vi "(Loop) HVPS_2.vi"   [LabVIEW 2017]
uses:
  Controls/(Ctrl) State_HVPS CMD.ctl
  Variables/(Var) System.vi
  Variables/(Var) Get_HVPS_2.vi
types:
  T1 = typedef "(Ctrl) State_HVPS CMD.ctl" = enum16{"Open", "Rx : V", "Rx : mA", "Rx : State", "Rx : ADC", "Tx : Set V", "Tx : Set mA", "Tx : ON", "Tx : OFF", "Close"}
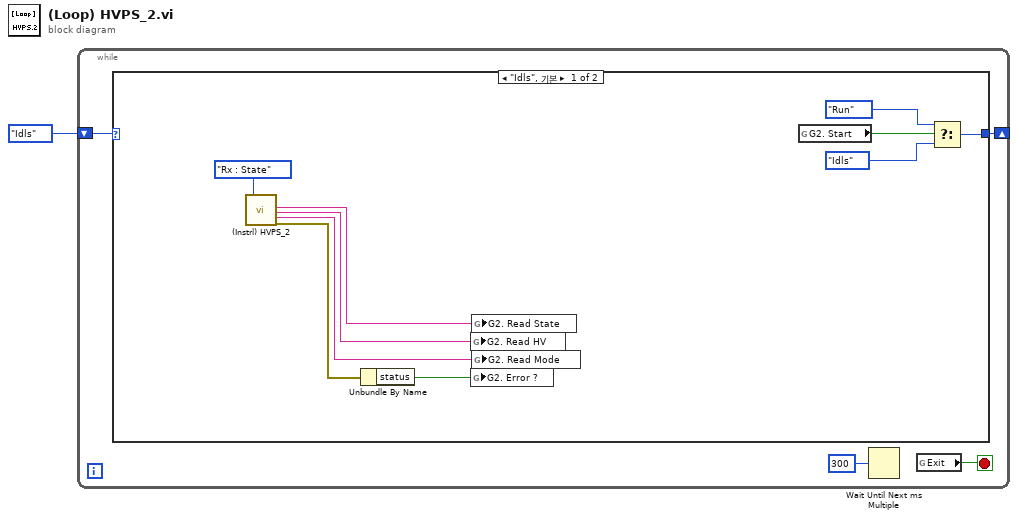
[diagram p0: block diagram]
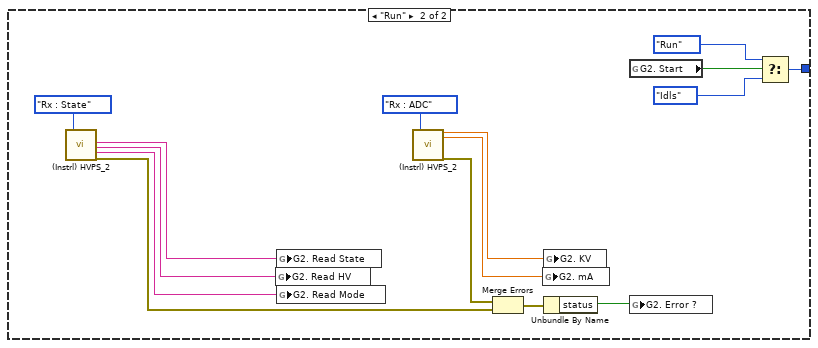
[diagram p2: hidden frame]
diagram:
  n1 = while {
    shift-right: [w2] -> _
    shift-left: enum16{"Init", "Idls", "Run", "Stop", "Close"}."Idls" -> [w4]
    stop <- w5 stop-if-true
    n2 = case shown="\"Idls\", 기본" w4 {
      tunnel: [w11 w27] -> w2
      frame "Idls", Default {
        n3 = call "(Instrl) HVPS_2.vi"("CMD"=(Ctrl)_State_HVPS_CMD."Rx : State" ("State")) -> ("System State"=w10:string, "HV State"=w9:string, "Operation Mode"=w8:string, "error out"=w14:errorcluster)  [unwired: 13 in, 2 out]
        n4 = Unbundle By Name(w14) -> ("status"=w7:bool)
        n5 = global write "(Var) Get_HVPS_2.vi" "G2. Read HV"(w9) -> ()
        n6 = global write "(Var) Get_HVPS_2.vi" "G2. Error ?"(w7) -> ()
        n7 = global write "(Var) Get_HVPS_2.vi" "G2. Read State"(w10) -> ()
        n8 = global write "(Var) Get_HVPS_2.vi" "G2. Read Mode"(w8) -> ()
        n9 = global read "(Var) Get_HVPS_2.vi" "G2. Start"() -> (w6:bool)
        n10 = Select(t=enum16{"Init", "Idls", "Run", "Stop", "Close"}."Run", s=w6, f=enum16{"Init", "Idls", "Run", "Stop", "Close"}."Idls") -> (s? t:f=w11:enum16{"Init", "Idls", "Run", "Stop", "Close"})
      }
      frame "Run" {
        n11 = call "(Instrl) HVPS_2.vi"("CMD"=(Ctrl)_State_HVPS_CMD."Rx : State" ("State")) -> ("System State"=w22:string, "HV State"=w21:string, "Operation Mode"=w20:string, "error out"=w23:errorcluster)  [unwired: 13 in, 2 out]
        n12 = global write "(Var) Get_HVPS_2.vi" "G2. Read HV"(w21) -> ()
        n13 = global write "(Var) Get_HVPS_2.vi" "G2. Read State"(w22) -> ()
        n14 = global write "(Var) Get_HVPS_2.vi" "G2. Read Mode"(w20) -> ()
        n15 = call "(Instrl) HVPS_2.vi"("CMD"=(Ctrl)_State_HVPS_CMD."Rx : ADC" ("State")) -> ("Get V"=w18:dbl, "Get mA"=w17:dbl, "error out"=w24:errorcluster)  [unwired: 13 in, 3 out]
        n16 = Merge Errors(w24, w23) -> (w25:errorcluster)
        n17 = global write "(Var) Get_HVPS_2.vi" "G2. mA"(w17) -> ()
        n18 = global write "(Var) Get_HVPS_2.vi" "G2. KV"(w18) -> ()
        n19 = Unbundle By Name(w25) -> ("status"=w19:bool)
        n20 = global read "(Var) Get_HVPS_2.vi" "G2. Start"() -> (w16:bool)
        n21 = global write "(Var) Get_HVPS_2.vi" "G2. Error ?"(w19) -> ()
        n22 = Select(t=enum16{"Init", "Idls", "Run", "Stop", "Close"}."Run", s=w16, f=enum16{"Init", "Idls", "Run", "Stop", "Close"}."Idls") -> (s? t:f=w27:enum16{"Init", "Idls", "Run", "Stop", "Close"})
      }
    }
    n23 = Wait Until Next ms Multiple(millisecond multiple=u32 300 ("대기 시간 (ms)")) -> ()  [unwired: 1 out]
    n24 = global read "(Var) System.vi" "Exit"() -> (w5:bool)
  }
